vi "Inficon - XML generator.vi"() -> ()   [LabVIEW 2016]
uses:
  Typedef/Inficon - Evaporator parameters.ctl
  <vilib>/Utility/xml.llb/Write to XML File(string).vi
panel:
  in  "Evaporator parameters":T1={"Rise Time 1 [mm:ss]"=0.0, "Soak Power 1 [%]"=0.0, "Soak Time 1 [mm:ss]"=0.0, "Rise Time 2 [mm:ss]"=0.0, "Soak Power 2 [%]"=0.0, "Soak Time 2 [mm:ss]"=0.0, "Shutter Delay"=enum."No", "New Rate"=0.0, "Rate Ramp Time [mm:ss]"=0.0, "Idle Ramp [mm:ss]"=0.0, "Idle Power [%]"=0.0, "Time Power"=enum."No", "Xtal Switch S"=0, "Xtal Switch Q"=0, "Tool Factor 1"=10.0, "Tool Factor 2"=10.0, "Deposition Rate [Å/s]"=0.0, "Final Thickness [kÅ]"=0.0, "Thickness Spt [kÅ]"=0.0, "Density [g/cm3]"=0.5, "Z-Ratio"=0.1, "Sensor"=1, "Source"=1, "Crucible"=1, "Control Gain [%]"=0.1, "Control TC [s]"=0.1, "Control DT [s] 2"=0.1, "Max Power"=0.1, "Sample"=1, "Hold Time [mm:ss]"=0.0} {"Hold Time [mm:ss]" min=0.0 max=5999.0 format="%<%M:%S>t"; "Sample" max=99 step=1; "Max Power" min=0.0 max=100.0 step=0.1 format="%.;%.1f"; "Control DT [s] 2" min=0.1 max=100.0 step=0.1 format="%.;%.1f"; "Control TC [s]" min=0.1 max=100.0 step=0.1 format="%.;%.1f"; "Control Gain [%]" min=0.01 max=99.99 step=0.01 format="%.;%.3f"; "Crucible" max=8 step=1; "Source" min=1 max=2 step=1; "Sensor" min=1 max=2 step=1; "Z-Ratio" min=0.1 max=9.999 step=0.001 format="%.;%.3f"; "Density [g/cm3]" min=0.5 max=99.99 step=0.01 format="%.;%.2f"; "Thickness Spt [kÅ]" min=0.0 max=999.0 step=0.001 format="%.;%.3f"; "Final Thickness [kÅ]" min=0.0 max=999.0 step=0.001 format="%.;%.3f"; "Deposition Rate [Å/s]" min=0.0 max=999.9 step=0.1 format="%.;%.1f"; "Tool Factor 2" min=10.0 max=500.0 step=0.1 format="%.;%.1f"; "Tool Factor 1" min=10.0 max=500.0 step=0.1 format="%.;%.1f"; "Xtal Switch Q" max=9 step=1; "Xtal Switch S" max=9 step=1; "Idle Power [%]" min=0.0 max=100.0 step=0.1 format="%.;%.1f"; "Idle Ramp [mm:ss]" min=0.0 max=5999.0 format="%<%M:%S>t"; "Rate Ramp Time [mm:ss]" min=0.0 max=5999.0 format="%<%M:%S>t"; "New Rate" min=0.0 max=999.9 step=0.1 format="%.;%.1f"; "Soak Time 2 [mm:ss]" min=0.0 max=5999.0 format="%<%M:%S>t"; "Soak Power 2 [%]" min=0.0 max=100.0 step=0.1 format="%.;%.1f"; "Soak Time 1 [mm:ss]" min=0.0 max=5999.0 format="%<%M:%S>t"; "Rise Time 2 [mm:ss]" min=0.0 max=5999.0 format="%<%M:%S>t"; "Soak Power 1 [%]" min=0.0 max=100.0 step=0.1 format="%.;%.1f"; "Rise Time 1 [mm:ss]" min=0.0 max=5999.0 format="%<%M:%S>t"}
  in  "Metal name":string
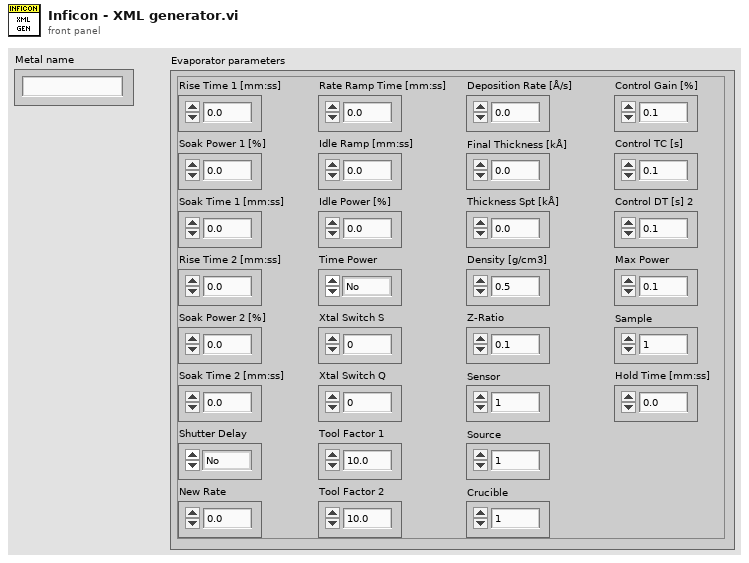
[diagram p1: front panel]
types:
  T1 = typedef "Inficon - Evaporator parameters.ctl" = cluster{"Rise Time 1 [mm:ss]":dbl, "Soak Power 1 [%]":dbl, "Soak Time 1 [mm:ss]":dbl, "Rise Time 2 [mm:ss]":dbl, "Soak Power 2 [%]":dbl, "Soak Time 2 [mm:ss]":dbl, "Shutter Delay":enum16{"No", "Yes"}, "New Rate":dbl, "Rate Ramp Time [mm:ss]":dbl, "Idle Ramp [mm:ss]":dbl, "Idle Power [%]":dbl, "Time Power":enum16{"No", "Yes"}, "Xtal Switch S":u8, "Xtal Switch Q":u8, "Tool Factor 1":dbl, "Tool Factor 2":dbl, "Deposition Rate [Å/s]":dbl, "Final Thickness [kÅ]":dbl, "Thickness Spt [kÅ]":dbl, "Density [g/cm3]":dbl, "Z-Ratio":dbl, "Sensor":u8, "Source":u8, "Crucible":u8, "Control Gain [%]":dbl, "Control TC [s]":dbl, "Control DT [s] 2":dbl, "Max Power":dbl, "Sample":u8, "Hold Time [mm:ss]":dbl}
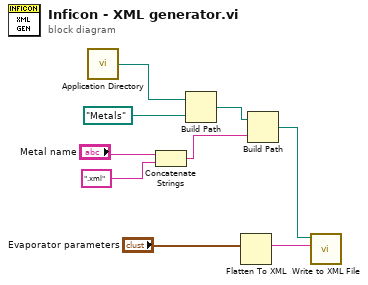
[diagram p0: block diagram]
diagram:
  n1 = call <vilib>:"Application Directory.vi"() -> ("Application Directory"=w8:path)
  n2 = Concatenate Strings("Metal name", ".xml" ("string")) -> (w2:string)
  n3 = Build Path(base path=w8, name or relative path=path "Metals") -> (appended path=w5:path)
  n4 = Flatten To XML(anything="Evaporator parameters") -> (xml string=w9:string)
  n5 = Build Path(base path=w5, name or relative path=w2) -> (appended path=w4:path)
  n6 = call-poly <vilib>:"Write to XML File.vi"("XML Input"=w9, "XML File Path"=w4) -> ()  [unwired: 7 in, 3 out]
